vi "Delete Item from Targets.vi"(7 "Type":string, 8 "error in (no error)":errorcluster, 9 "Item Name":string, 10 "Target Names in":string[](array[string]), 11 "Project Sync Tools in":refnum<class "Project Sync Tools.lvclass">) -> (0 "error out":errorcluster, 2 "Target Names out":string[](array[string]), 3 "Project Sync Tools out":refnum<class "Project Sync Tools.lvclass">)   [LabVIEW 2019, in "Project Sync Tools.lvclass"]
uses:
  Project Sync Tools.lvclass
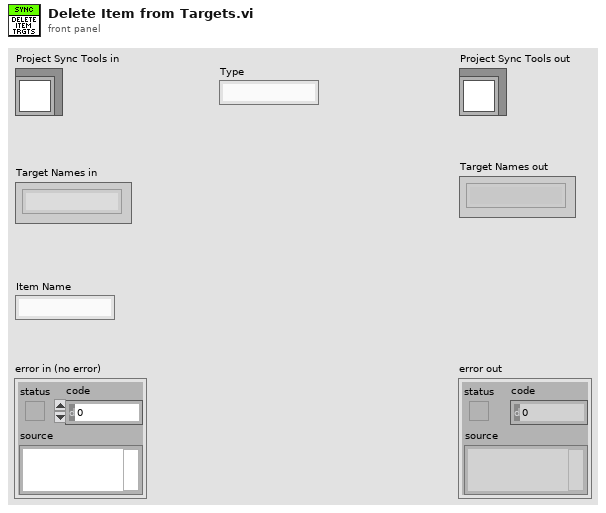
[diagram p1: front panel]
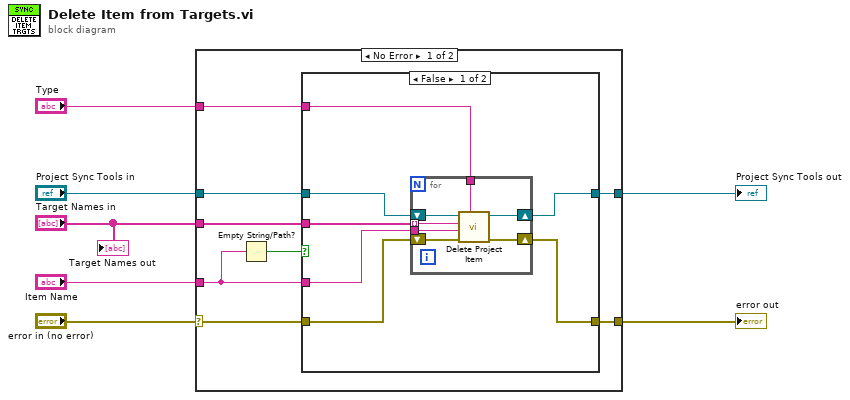
[diagram p0: block diagram]
diagram:
  n1 = case shown="No Error" "error in (no error)" {
    selector: "error in (no error)" -> [w13 w33]
    tunnel: [w12 w33] -> w6
    tunnel: [w14 w32] -> w4
    tunnel: "Project Sync Tools in" -> [w15 w32]
    tunnel: "Type" -> [w11 _]
    tunnel: "Target Names in" -> [w10 _]
    tunnel: "Item Name" -> [w8 _]
    frame No Error {
      n2 = Empty String/Path?(string/path=w8) -> (empty?=w9:bool)
      n3 = case shown="False" w9 {
        tunnel: w15 -> [w22 w31]
        tunnel: [w21 w31] -> w14
        tunnel: w13 -> [w20 w30]
        tunnel: [w19 w30] -> w12
        tunnel: w11 -> [w18 _]
        tunnel: w10 -> [w17 _]
        tunnel: w8 -> [w16 _]
        frame False {
          n4 = for {
            shift-right: [w27] -> w21
            shift-left: w22 -> [w28]
            shift-right: [w26] -> w19
            shift-left: w20 -> [w29]
            tunnel: w18 -> [w25]
            tunnel: w17 -> [w24] mode=indexing
            tunnel: w16 -> [w23]
            n5 = call "Delete Project Item.vi"("Type"=w25, "error in (no error)"=w29, "Item Name"=w23, "Target Name"=w24, "Project Sync Tools in"=w28) -> ("error out"=w26:errorcluster, "Project Sync Tools out"=w27:refnum<class "Project Sync Tools.lvclass">)  [unwired: 5 in]
          }
        }
        frame True {
        }
      }
    }
    frame Error {
    }
  }
  "error out" <- w6
  "Project Sync Tools out" <- w4
  "Target Names out" <- "Target Names in"
